vi "DT_Subset.vi"(10 "Subset":cluster{"start idx":i32, "length":i32}[](array[cluster]), 11 "Points In":cluster{"x":dbl, "y":dbl, "index":i32}[](array[cluster])) -> (0 "error":i32, 1 "Subset Triangles":cluster{"Triangles":i32[][]}[](array[cluster]), 2 "Subset Out":cluster{"start idx":i32, "length":i32}[](array[cluster]), 3 "Points Out":cluster{"x":dbl, "y":dbl, "index":i32}[](array[cluster]))   [LabVIEW 2020, in "NI_AAL_Geometry.lvlib"]
uses:
  <vilib>/Analysis/NI_AAL_Geometry.lvlib
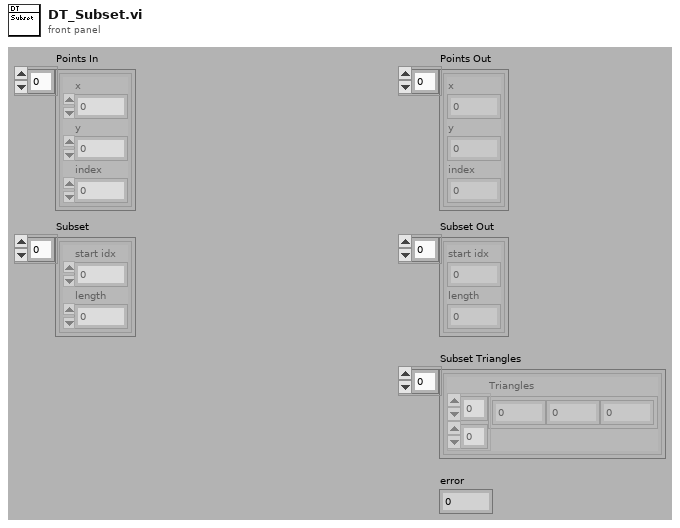
[diagram p1: front panel]
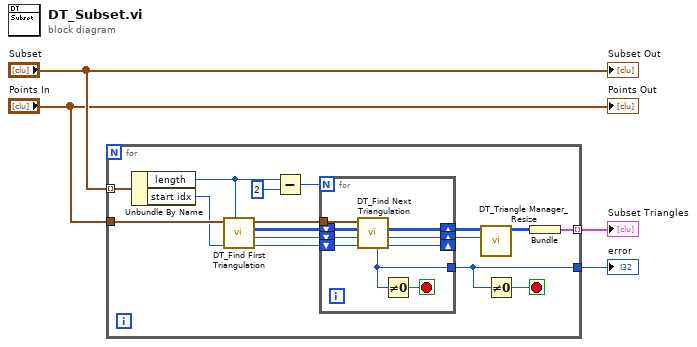
[diagram p0: block diagram]
diagram:
  n1 = for {
    tunnel: [w19] -> w4 mode=indexing
    tunnel: "Points In" -> [w10]
    tunnel: "Subset" -> [w17] mode=indexing
    tunnel: [w5] -> w1
    stop <- w6 stop-if-true
    n2 = Unbundle By Name(w17) -> ("length"=w8:i32, "start idx"=w7:i32)
    n3 = call <vilib>:"DT_Find First Triangulation.vi"("length"=w8, "cur point"=w7, "Points In"=w10) -> ("next point"=w11:i32, "next triangle"=w12:i32, "Triangles"=w13:i32[][], "Points Out"=w18:cluster{"x":dbl, "y":dbl, "index":i32}[])  [unwired: 5 out]
    n4 = Subtract(x=w8, y=2) -> (x-y=w20:i32)
    n5 = for {
      N: w20 -> [_]
      shift-right: [w27] -> w16
      shift-left: w13 -> [w28]
      shift-right: [w25] -> w14
      shift-left: w12 -> [w26]
      tunnel: w18 -> [w29]
      shift-right: [w23] -> _
      shift-left: w11 -> [w24]
      tunnel: [w21] -> w5
      stop <- w22 stop-if-true
      n6 = call <vilib>:"DT_Find Next Triangulation.vi"("cur point"=w24, "next triangle in"=w26, "Triangles In"=w28, "Points In"=w29) -> ("next point"=w23:i32, "next triangle out"=w25:i32, "Triangles Out"=w27:i32[][], "error"=w21:i32)  [unwired: 1 in, 3 out]
      n7 = Not Equal To 0?(x=w21) -> (x != 0?=w22:bool)
    }
    n8 = call <vilib>:"DT_Triangle Manager_Resize.vi"("# of triangles"=w14, "Triangles In"=w16) -> ("Triangles Out"=w15:i32[][])  [unwired: 9 out]
    n9 = Not Equal To 0?(x=w5) -> (x != 0?=w6:bool)
    n10 = Bundle("Triangles Out"=w15) -> (w19:cluster{"Triangles Out":i32[][]})  [unwired: 1 in]
  }
  "Subset Triangles" <- w4
  "error" <- w1
  "Points Out" <- "Points In"
  "Subset Out" <- "Subset"
